vi "slv addr format fgv.vi"(7 "function":T2, 8 "error in (no error)":errorcluster caption="에러 입력(에러 없음)", 11 "i2c slv addr format in":T1) -> (0 "error out":errorcluster caption="에러 출력", 3 "i2c slv addr format out":T1)   [LabVIEW 2020, in "I2C.lvclass"]
uses:
  I2C.lvclass
  Controls/(Ctrl)i2c slv addr format fgv enum.ctl
  Controls/(Ctrl)i2c slv addr format.ctl
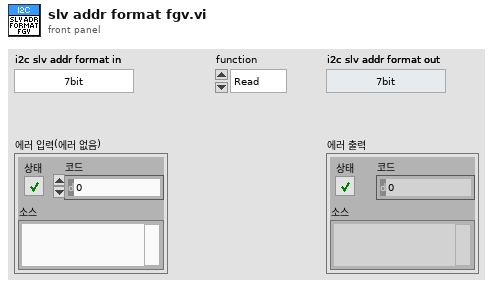
[diagram p1: front panel]
types:
  T1 = typedef "I2C.lvclass/(Ctrl)i2c slv addr format.ctl" = enum16{"7bit", "8bit"}
  T2 = typedef "I2C.lvclass/(Ctrl)i2c slv addr format fgv enum.ctl" = enum16{"Read", "Write"}
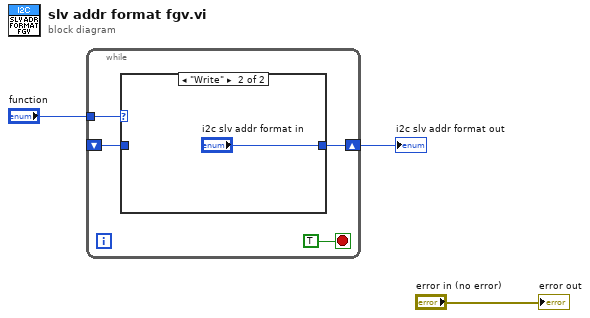
[diagram p0: block diagram]
diagram:
  n1 = while {
    shift-right: [w7] -> w2
    shift-left: _ -> [w4]
    tunnel: "function" -> [w5]
    stop <- TRUE stop-if-true
    n2 = case shown="\"Write\"" w5 {
      tunnel: [w8 "i2c slv addr format in"] -> w7
      tunnel: w4 -> [w8 _]
      frame "Read", Default {
      }
      frame "Write" {
      }
    }
  }
  "i2c slv addr format out" <- w2
  "error out" <- "error in (no error)"
